vi "Task 1.vi"() -> ()   [LabVIEW 2019]
panel:
  out "Max Temp String":string
  out "Min Temp String":string
  out "Max Temp LED":bool
  out "Min Temp LED":bool
  in  "Maximum Temperature":dbl
  in  "Minimum Temperature":dbl
  out "Current Temp Celcius":dbl
  in  "Current Temp Farheneit":dbl
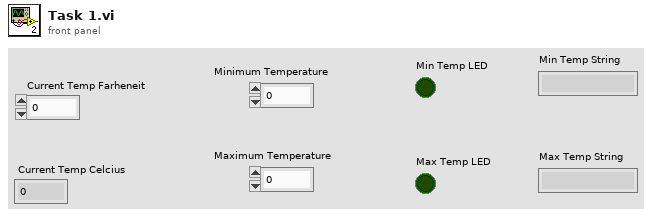
[diagram p1: front panel]
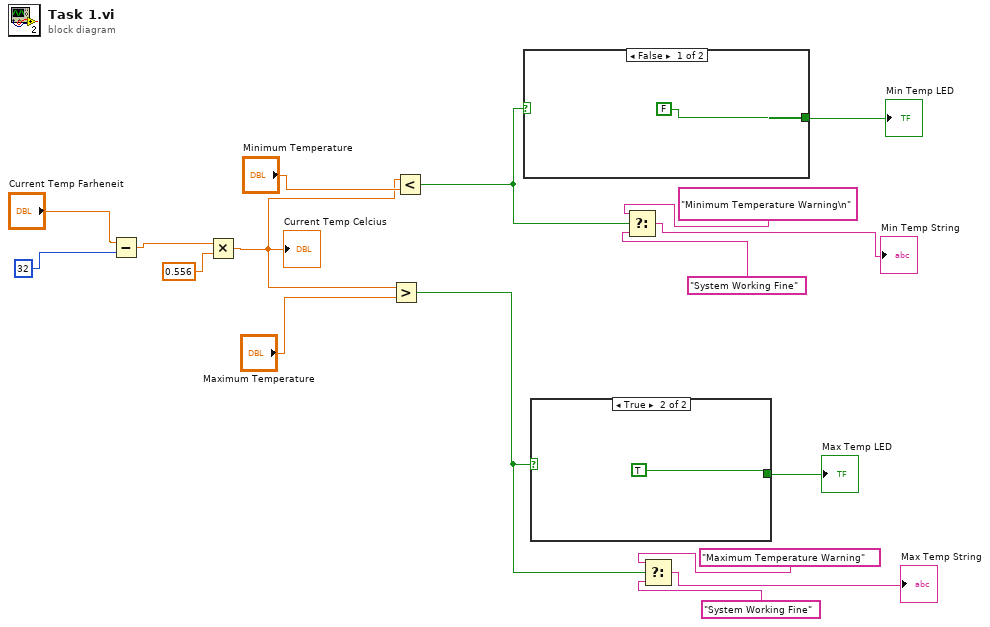
[diagram p0: block diagram]
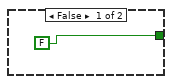
[diagram p2: hidden frame]
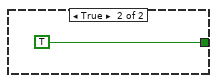
[diagram p3: hidden frame]
diagram:
  n1 = Subtract(x="Current Temp Farheneit", y=32) -> (x-y=w15:dbl)
  n2 = Multiply(x=w15, y=0.556) -> (x*y=w11:dbl)
  "Current Temp Celcius" <- w11
  n3 = Greater?(x=w11, y="Maximum Temperature") -> (0:w9:bool)
  n4 = Less?(x=w11, y="Minimum Temperature") -> (x < y?=w10:bool)
  n5 = case shown="False" w10 {
    tunnel: [FALSE TRUE] -> w4
    frame False {
    }
    frame True {
    }
  }
  "Min Temp LED" <- w4
  n6 = case shown="True" w9 {
    tunnel: [FALSE TRUE] -> w3
    frame False {
    }
    frame True {
    }
  }
  "Max Temp LED" <- w3
  n7 = Select(t="Minimum Temperature Warning\n", s=w10, f="System Working Fine") -> (s? t:f=→"Min Temp String":string)
  n8 = Select(t="Maximum Temperature Warning", s=w9, f="System Working Fine") -> (s? t:f=→"Max Temp String":string)
